vi "GlobalMainVI.vi"() -> ()   [LabVIEW 2020]
panel:
  in  "User/Edit Tab Ref":refnum<vi>
  in  "MainTab Ref":refnum<vi>
  in  "MainVI Ref":refnum<vi>
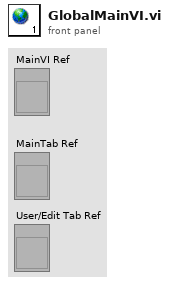
[diagram p1: front panel]
diagram:
